vi "Cali-Gauss.vi"() -> ()   [LabVIEW 2014]
uses:
  <vilib>/Analysis/6fits.llb/Curve Fitting Criteria.ctl
  <vilib>/vision/NI_Vision_Development_Module.lvlib
  <vilib>/Analysis/NI_AALPro.lvlib
  <vilib>/Analysis/NI_AALBase.lvlib
panel:
  out "Histogram Graph 2":T1(graph)
  out "XY Graph 3":cluster{dbl[], "Best Gaussian Fit":dbl[]}[](graph)=[{[101.48688930524672, 103.97785917958191, 106.4688290539171, 108.9597989282523, 111.45076880258749, 113.94173867692268, 116.43270855125787, 118.92367842559307, 121.41464829992826, 123.90561817426345, 126.39658804859864, 128.88755792293384, 131.37852779726902, 133.86949767160422, 136.3604675459394, 138.8514374202746, 141.34240729460979, 143.833377168945, 146.32434704328017, 148.81531691761538, 151.30628679195058, 153.79725666628576, 156.28822654062097, 158.77919641495615, 161.27016628929135, 163.76113616362653, 166.25210603796174, 168.74307591229692, 171.23404578663212, 173.7250156609673, 176.2159855353025, 178.7069554096377, 181.1979252839729, 183.68889515830807, 186.17986503264328, 188.67083490697846, 191.16180478131366, 193.65277465564884, 196.14374452998405, 198.63471440431923, 201.12568427865443, 203.6166541529896, 206.10762402732482, 208.59859390166, 211.0895637759952, 213.58053365033038, 216.0715035246656, 218.56247339900077, 221.05344327333597, 223.54441314767115, 226.03538302200636, 228.52635289634154, 231.01732277067674, 233.50829264501192, 235.99926251934713, 238.4902323936823, 240.9812022680175, 243.4721721423527, 245.9631420166879, 248.4541118910231, 250.94508176535828, 253.4360516396935, 255.92702151402867, 258.4179913883639, 260.90896126269905, 263.39993113703423, 265.89090101136946, 268.38187088570464, 270.8728407600398, 273.363810634375, 275.85478050871023, 278.3457503830454, 280.8367202573806, 283.32769013171577, 285.818660006051, 288.3096298803862, 290.80059975472136, 293.29156962905654, 295.7825395033918, 298.27350937772695], "Best Gaussian Fit"=[15.0, 11.0, 2.0, 5.0, 3.0, 2.0, 7.0, 8.0, 10.0, 12.0, 10.0, 10.0, 11.0, 16.0, 10.0, 12.0, 6.0, 3.0, 1.0, 1.0, 1.0, 1.0, 1.0, 0.0, 2.0, 4.0, 19.0, 57.0, 96.0, 131.0, 193.0, 224.0, 233.0, 166.0, 132.0, 111.0, 63.0, 43.0, 38.0, 27.0, 20.0, 24.0, 25.0, 19.0, 18.0, 13.0, 12.0, 6.0, 3.0, 2.0, 0.0, 3.0, 6.0, 2.0, 1.0, 0.0, 1.0, 3.0, 3.0, 2.0, 1.0, 4.0, 1.0, 5.0, 2.0, 2.0, 3.0, 3.0, 5.0, 4.0, 8.0, 3.0, 6.0, 5.0, 9.0, 7.0, 8.0, 15.0, 8.0, 13.0]}, {[101.48688930524672, 103.97785917958191, 106.4688290539171, 108.9597989282523, 111.45076880258749, 113.94173867692268, 116.43270855125787, 118.92367842559307, 121.41464829992826, 123.90561817426345, 126.39658804859864, 128.88755792293384, 131.37852779726902, 133.86949767160422, 136.3604675459394, 138.8514374202746, 141.34240729460979, 143.833377168945, 146.32434704328017, 148.81531691761538, 151.30628679195058, 153.79725666628576, 156.28822654062097, 158.77919641495615, 161.27016628929135, 163.76113616362653, 166.25210603796174, 168.74307591229692, 171.23404578663212, 173.7250156609673, 176.2159855353025, 178.7069554096377, 181.1979252839729, 183.68889515830807, 186.17986503264328, 188.67083490697846, 191.16180478131366, 193.65277465564884, 196.14374452998405, 198.63471440431923, 201.12568427865443, 203.6166541529896, 206.10762402732482, 208.59859390166, 211.0895637759952, 213.58053365033038, 216.0715035246656, 218.56247339900077, 221.05344327333597, 223.54441314767115, 226.03538302200636, 228.52635289634154, 231.01732277067674, 233.50829264501192, 235.99926251934713, 238.4902323936823, 240.9812022680175, 243.4721721423527, 245.9631420166879, 248.4541118910231, 250.94508176535828, 253.4360516396935, 255.92702151402867, 258.4179913883639, 260.90896126269905, 263.39993113703423, 265.89090101136946, 268.38187088570464, 270.8728407600398, 273.363810634375, 275.85478050871023, 278.3457503830454, 280.8367202573806, 283.32769013171577, 285.818660006051, 288.3096298803862, 290.80059975472136, 293.29156962905654, 295.7825395033918, 298.27350937772695], "Best Gaussian Fit"=[8.90785846088077e-29, 7.021130037433218e-27, 4.808229222350119e-25, 2.8609334048924016e-23, 1.479022469530185e-21, 6.643336229243675e-20, 2.5926394964550686e-18, 8.791084823183834e-17, 2.589925348785984e-15, 6.62943413638216e-14, 1.4743823129188916e-12, 2.848972141664502e-11, 4.783113989371778e-10, 6.977144177656755e-09, 8.842785737783608e-08, 9.737443368863115e-07, 9.316337771562747e-06, 7.744438671802883e-05, 0.0005593441524087933, 0.003510045106885543, 0.01913774356761686, 0.09065947560963374, 0.37314713586253756, 1.3344166753364568, 4.146171351529102, 11.193024921297205, 26.253797617721034, 53.50338181819122, 94.73594077343999, 145.74469275032772, 194.8117573100726, 226.24657686947603, 228.2933748097909, 200.1469782119382, 152.4576443327255, 100.90061439539565, 58.020685355062504, 28.98787209696965, 12.583291472450126, 4.745878490205033, 1.5551898424014134, 0.4427867795631612, 0.10953434565087419, 0.02354238344273649, 0.004396377513090009, 0.0007133192838737798, 0.00010055817667299242, 1.2316725242603104e-05, 1.3107430237470307e-06, 1.2119488600908989e-07, 9.7363341923314e-09, 6.795964290823915e-10, 4.1214605031981886e-11, 2.171679013453158e-12, 9.942247377031198e-14, 3.954739969994927e-15, 1.3667709511385086e-16, 4.1041004767105474e-18, 1.0707415790851268e-19, 2.427145370573475e-21, 4.780258118819467e-23, 8.179963110116992e-25, 1.2161741847293132e-26, 1.5710306362369438e-28, 1.7632665382810075e-30, 1.7194744059961332e-32, 1.456860283532724e-34, 1.0724684626474922e-36, 6.859549499215879e-39, 3.8119842432472027e-41, 1.8405644836287736e-43, 7.721388708643295e-46, 2.8143897023271556e-48, 8.91286827584324e-51, 2.452421874936481e-53, 5.8629651482181345e-56, 1.2178221870196085e-58, 2.1978340105667308e-61, 3.446278219981271e-64, 4.6951580827582554e-67]}]
  out "center":dbl
  out "Histogram Graph":T1(graph)
  out "dis":dbl[][](array[numeric])
  out "y mesh":i32[][](array[numeric])
  out "x mesh":i32[][](array[numeric])
  out "element":i32
  out "Image Pixels (U8) 2":u8[](array[numeric])
  out "Image Pixels (U8)":u8[][](array[numeric])
  in  "Optional Rectangle":i32[](array[numeric])=[1400, 0]
  out "Image 2":T2(plugin-control)
  in  "File Path":path=path "C:/Users/OT-hwLi-lab/Desktop/YCC/NewTPM/4.Other/cal.png"
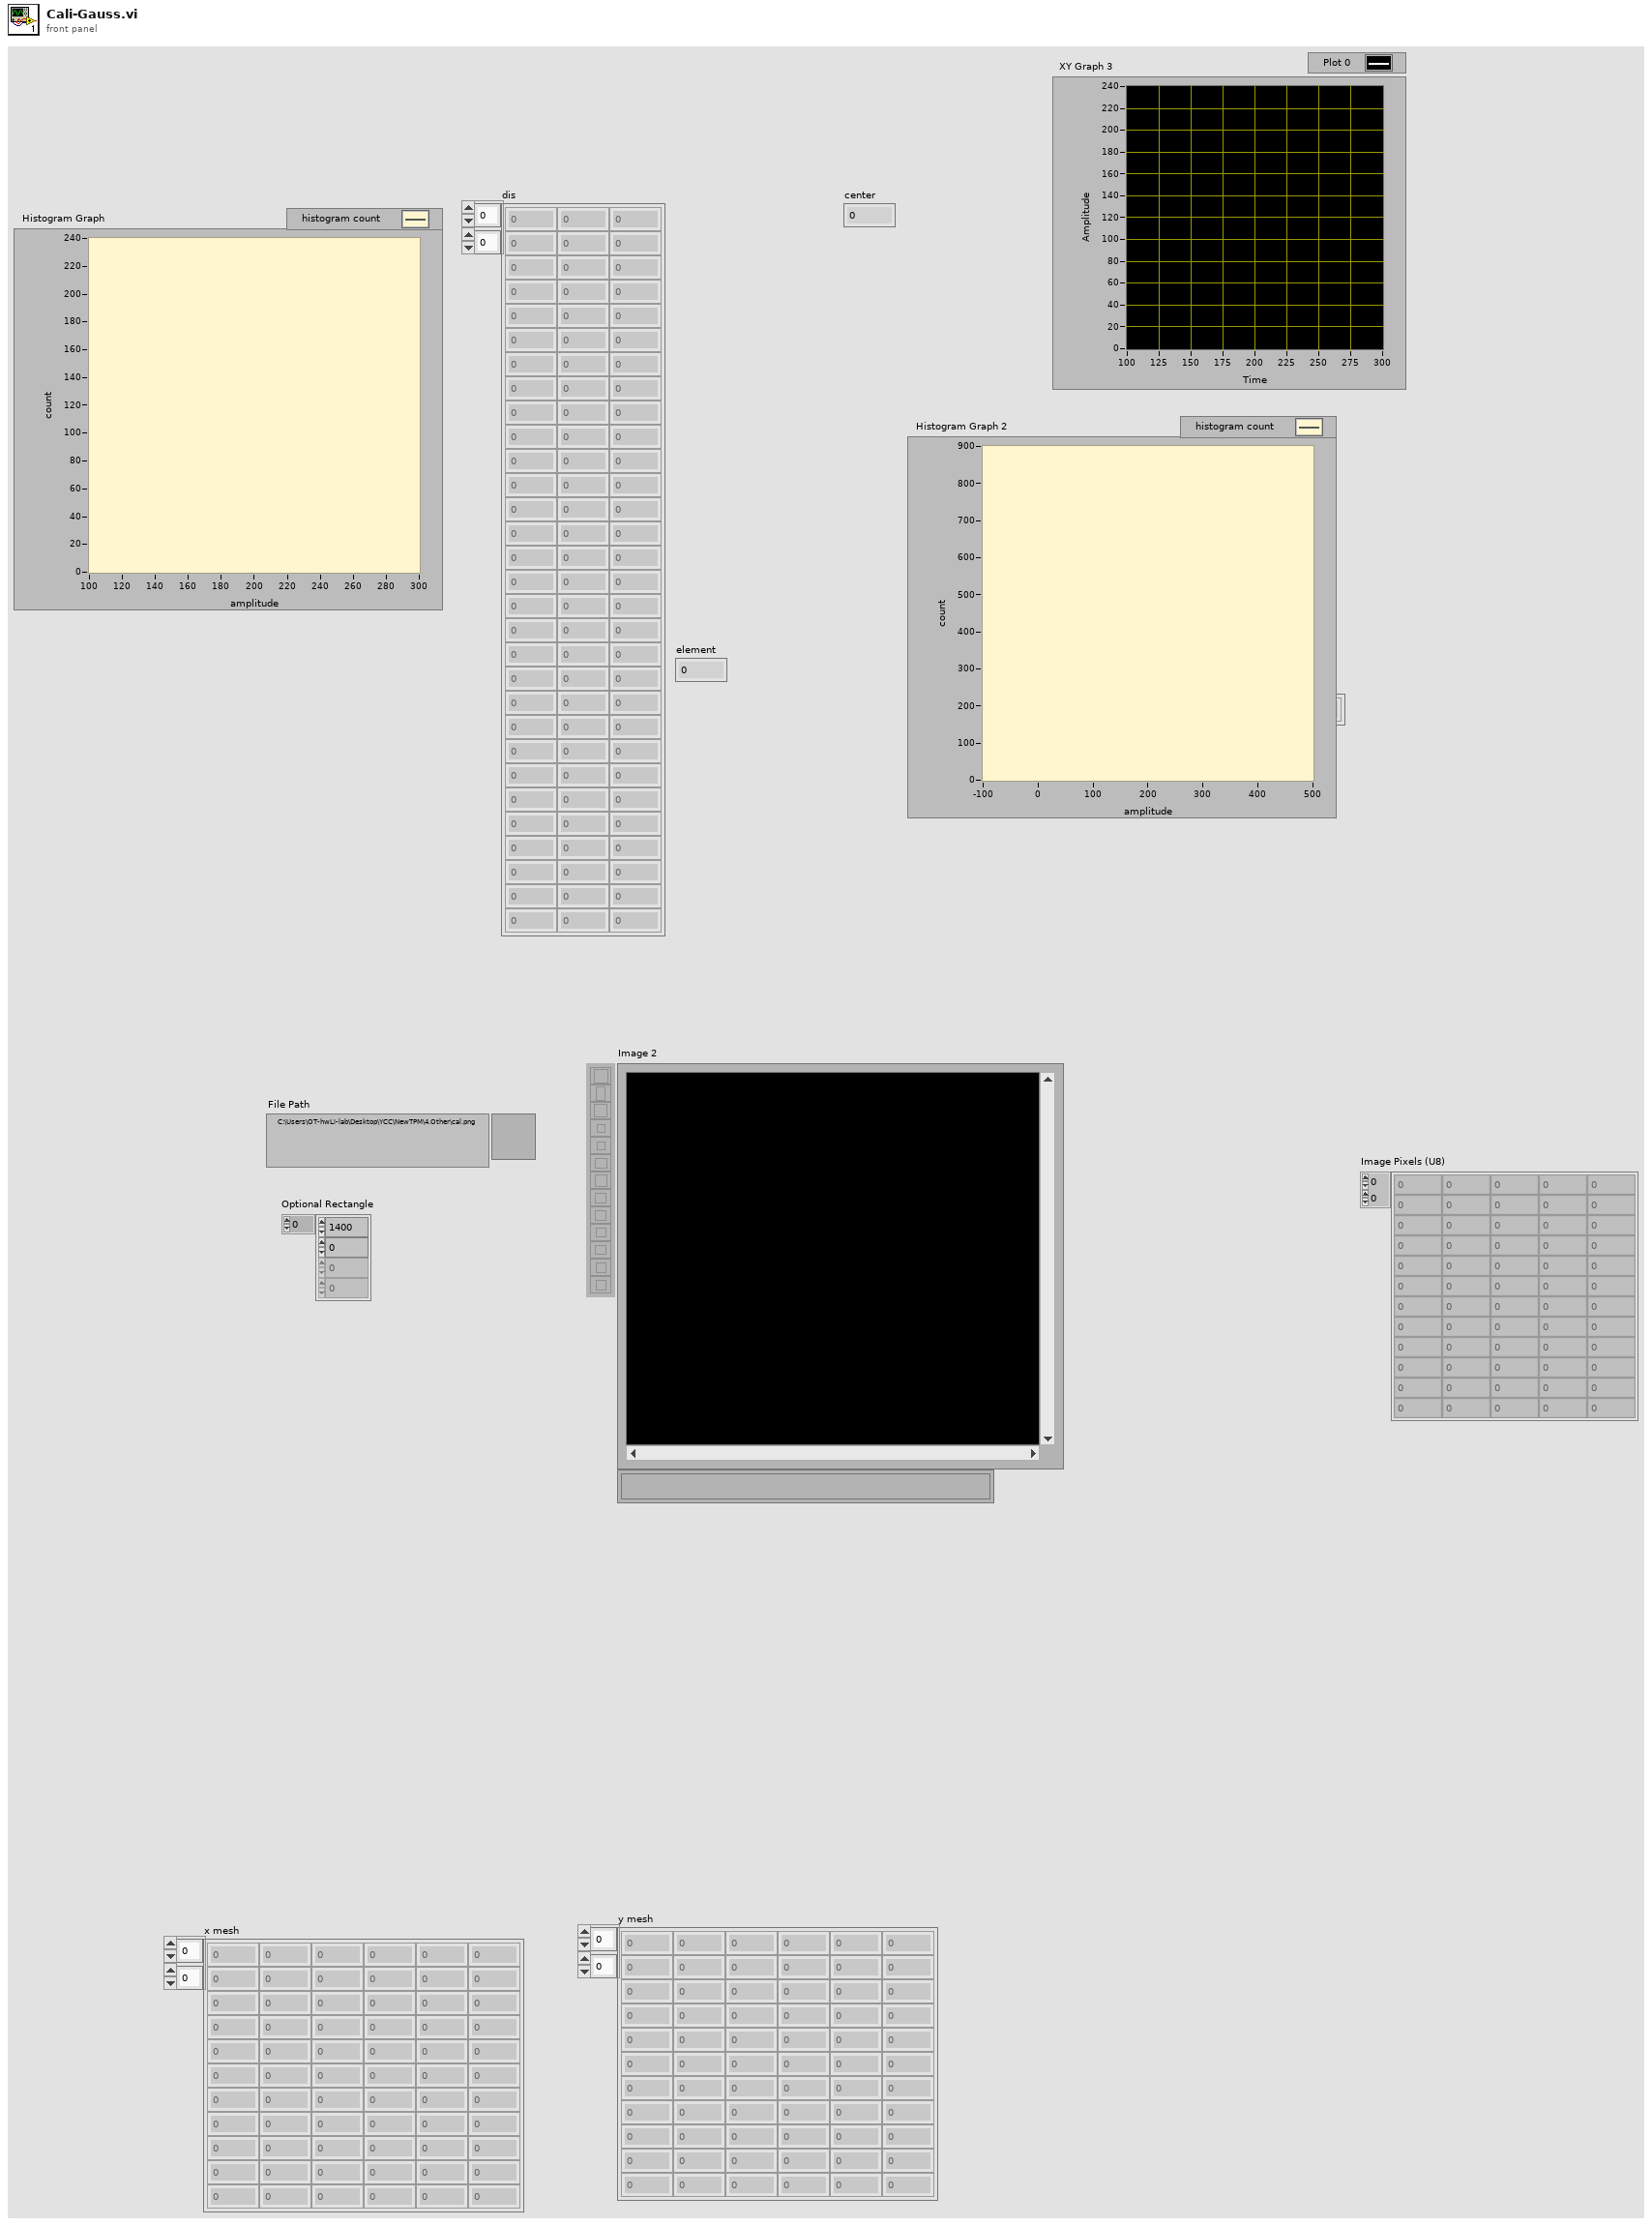
[diagram p1: front panel]
types:
  T1 = cluster{"X Values":dbl[], "Histogram: h(x)":i32[]}
  T2 = typedef "IMAQ Image.ctl" = refnum<image>
  T3 = typedef "Image Type" = u32
  T4 = typedef "NI_AALPro.lvlib/Curve Fitting Criteria.ctl" = u16
  T5 = cluster{"X Values":dbl[], "Best Gaussian Fit":dbl[]}
  T6 = cluster{"X Values":dbl[], "Best Gaussian Fit":dbl[]}[]
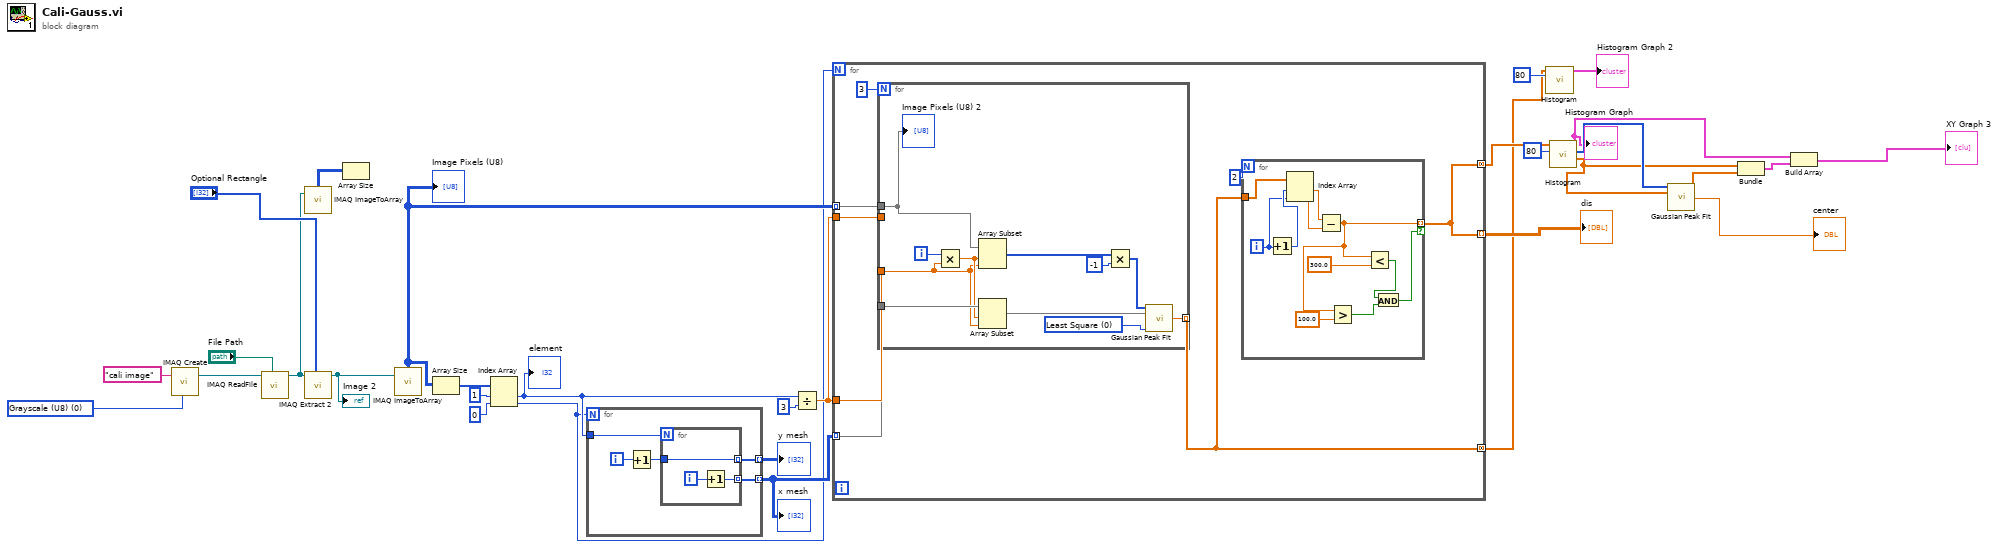
[diagram p0: block diagram]
diagram:
  w29 = T3 0 items=["Grayscale (U8)", "Grayscale (I16)", "Grayscale (SGL)", "Complex (CSG)", "RGB (U32)", "HSL (U32)", "RGB (U64)", "Grayscale (U16)"] ("Image Type")
  n1 = call "IMAQ Create"("Image Name"="cali image", "Image Type"=w29) -> ("New Image"=w28:T2)  [unwired: 3 in, 1 out]
  n2 = call "IMAQ ReadFile"("File Path"="File Path", "Image"=w28) -> ("Image Out"=w26:T2)  [unwired: 5 in, 4 out]
  n3 = call "IMAQ ImageToArray"("Image"=w26) -> ("Image Pixels (U8)"=w25:u8[][])  [unwired: 3 in, 4 out]
  n4 = call "IMAQ Extract 2"("Optional Rectangle"="Optional Rectangle", "Image Src"=w26) -> ("Image Dst Out"=w24:T2)  [unwired: 8 in, 1 out]
  "Image 2" <- w24
  n5 = Array Size(array=w25) -> ()  [unwired: 1 out]
  n6 = call "IMAQ ImageToArray"("Image"=w24) -> ("Image Pixels (U8)"=w23:u8[][])  [unwired: 3 in, 4 out]
  "Image Pixels (U8)" <- w23
  n7 = Array Size(array=w23) -> (size(s)=w22:i32[])
  n8 = Index Array(array=w22, index #1=1 ("index"), index #2=0 ("index")) -> (element #1=w17:i32, element #2=w14:i32)
  "element" <- w17
  n9 = for {
    N: w14 -> [_]
    tunnel: [w34] -> w18 mode=indexing
    tunnel: [w33] -> w16 mode=indexing
    tunnel: w17 -> [w32]
    i -> [w36]
    n10 = Increment(x=w36) -> (x+1=w35:i32)
    n11 = for {
      N: w32 -> [_]
      tunnel: w35 -> [w39]
      tunnel: [w39] -> w34 mode=indexing
      tunnel: [w37] -> w33 mode=indexing
      i -> [w38]
      n12 = Increment(x=w38) -> (x+1=w37:i32)
    }
  }
  "x mesh" <- w16
  "y mesh" <- w18
  n13 = Divide(x=w17, y=3) -> (x/y=w15:dbl)
  n14 = for {
    N: w14 -> [_]
    tunnel: w23 -> [w47] mode=indexing
    tunnel: w15 -> [w46]
    tunnel: w16 -> [w45] mode=indexing
    tunnel: w15 -> [w43]
    tunnel: [w42] -> w1 mode=concatenating
    tunnel: [w40] -> w13 mode=indexing
    tunnel: [w40] -> w3 mode=concatenating
    n15 = for {
      N: 3 -> [_]
      tunnel: w47 -> [w69]
      tunnel: w46 -> [w66]
      tunnel: w45 -> [w68]
      tunnel: w43 -> [_]
      tunnel: [w61] -> w42 mode=indexing
      i -> [w60]
      w59 = T4 0 items=["Least Square", "Least Absolute Residual", "Bisquare"] ("method")
      n16 = Multiply(x=w60, y=w66) -> (x*y=w67:dbl)
      n17 = Array Subset "Array Subset"(array=w69, index=w67, length=w66) -> (w65:u8[])
      n18 = Array Subset "Array Subset"(array=w68, index=w67, length=w66) -> (w62:i32[])
      n19 = Multiply(x=w65, y=-1) -> (x*y=w63:i32[])
      n20 = call <vilib>:"Gaussian Peak Fit.vi"("Y"=w63, "X"=w62, "method"=w59) -> ("center"=w61:dbl)  [unwired: 6 in, 6 out]
      "Image Pixels (U8) 2" <- w69
    }
    n21 = for {
      N: 2 -> [_]
      tunnel: w42 -> [w58]
      tunnel: [w52] -> w40 mode=indexing if=w48
      i -> [w56]
      n22 = Increment(x=w56) -> (x+1=w57:i32)
      n23 = Index Array(array=w58, index #1=w57, index #2=w56) -> (element #1=w55:dbl, element #2=w54:dbl)
      n24 = Subtract(x=w55, y=w54) -> (x-y=w52:dbl)
      n25 = Greater?(x=w52, y=100.0) -> (0:w49:bool)
      n26 = Less?(x=w52, y=300.0) -> (x < y?=w50:bool)
      n27 = And(x=w50, y=w49) -> (x .and. y?=w48:bool)
    }
  }
  "dis" <- w13
  n28 = call <vilib>:"Histogram.vi"("intervals"=80, "X"=w1) -> ("Histogram Graph"=→"Histogram Graph 2":T1)  [unwired: 6 in, 3 out]
  n29 = call <vilib>:"Histogram.vi"("intervals"=80, "X"=w3) -> ("X Values"=w7:dbl[], "Histogram: h(x)"=w10:i32[], "Histogram Graph"=w5:T1)  [unwired: 6 in, 1 out]
  "Histogram Graph" <- w5
  n30 = call <vilib>:"Gaussian Peak Fit.vi"("Y"=w10, "X"=w7) -> ("Best Gaussian Fit"=w8:dbl[], "center"=→"center":dbl)  [unwired: 7 in, 5 out]
  n31 = Bundle("X Values"=w7, "Best Gaussian Fit"=w8) -> (w6:T5)  [unwired: 1 in]
  n32 = Build Array(w5, w6) -> (→"XY Graph 3":T6)
